vi "Tester.vi"(5 "port or service name":u16, 7 "IP":string, 8 "error in (no error)":errorcluster, 9 "timeout ms (25000)":i32=2000, 10 "Command":string, 11 "connection ID":refnum<k16>) -> (0 "error out":errorcluster, 1 "iteration":i32, 2 "checker":string, 3 "connection ID":refnum<k16>)   [LabVIEW 2018, in "Simple UDP Message.lvlib"]
uses:
  Simple UDP Message.lvlib
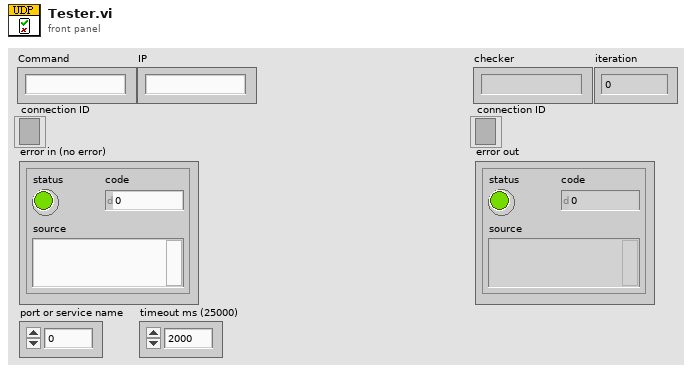
[diagram p1: front panel]
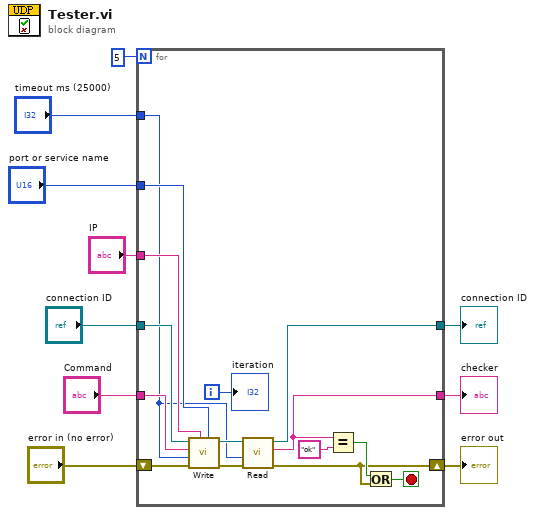
[diagram p0: block diagram]
diagram:
  n1 = for {
    N: 5 -> [_]
    tunnel: "Command" -> [w23]
    tunnel: [w20] -> w9
    tunnel: "connection ID" -> [w22]
    tunnel: [w21] -> w7
    tunnel: "IP" -> [w16]
    shift-right: [w14] -> w5
    shift-left: "error in (no error)" -> [w17]
    tunnel: "port or service name" -> [w12]
    tunnel: "timeout ms (25000)" -> [w11]
    i -> [w13]
    stop <- w15 stop-if-true
    n2 = call "Write.vi"("port or service name"=w12, "IP"=w16, "error in (no error)"=w17, "timeout ms (25000)"=w11, "data in"=w23, "connection ID"=w22) -> ("error out"=w25:errorcluster, "connection ID"=w24:refnum<k16>)  [unwired: 4 in]
    n3 = call "Read.vi"("error in (no error)"=w25, "timeout ms (25000)"=w11, "connection ID"=w24) -> ("error out"=w14:errorcluster, "data out"=w20:string, "connection ID"=w21:refnum<k16>)  [unwired: 4 in, 2 out]
    n4 = Equal?(x=w20, y="ok") -> (x = y?=w18:bool)
    n5 = Or(x=w18, y=w14) -> (x .or. y?=w15:bool)
    "iteration" <- w13
  }
  "checker" <- w9
  "connection ID" <- w7
  "error out" <- w5
